vi "samyoung_pm_ZOU.vi"() -> ()   [LabVIEW 2015]
uses:
  <vilib>/DAQmx/read.llb/DAQmx Read.vi
  <vilib>/DAQmx/read.llb/DAQmx Read (Analog DBL 1Chan 1Samp).vi
  <vilib>/DAQmx/create/channels.llb/DAQmx Create Channel (AI-Voltage-Basic).vi
  <vilib>/DAQmx/configure/timing.llb/DAQmx Timing (Sample Clock).vi
  <vilib>/Utility/file.llb/Write To Spreadsheet File (string).vi
  <vilib>/DAQmx/miscellaneous.llb/DAQmx Fill In Error Info.vi
panel:
  in  "Fille Directory":path
  in  "error in":errorcluster
  in  "samples per channel":i32=1000
  in  "rate":dbl=1000.0 format="%0.2f"
  in  "stop":bool
  # "Dust and Gas Sensor Module Output"
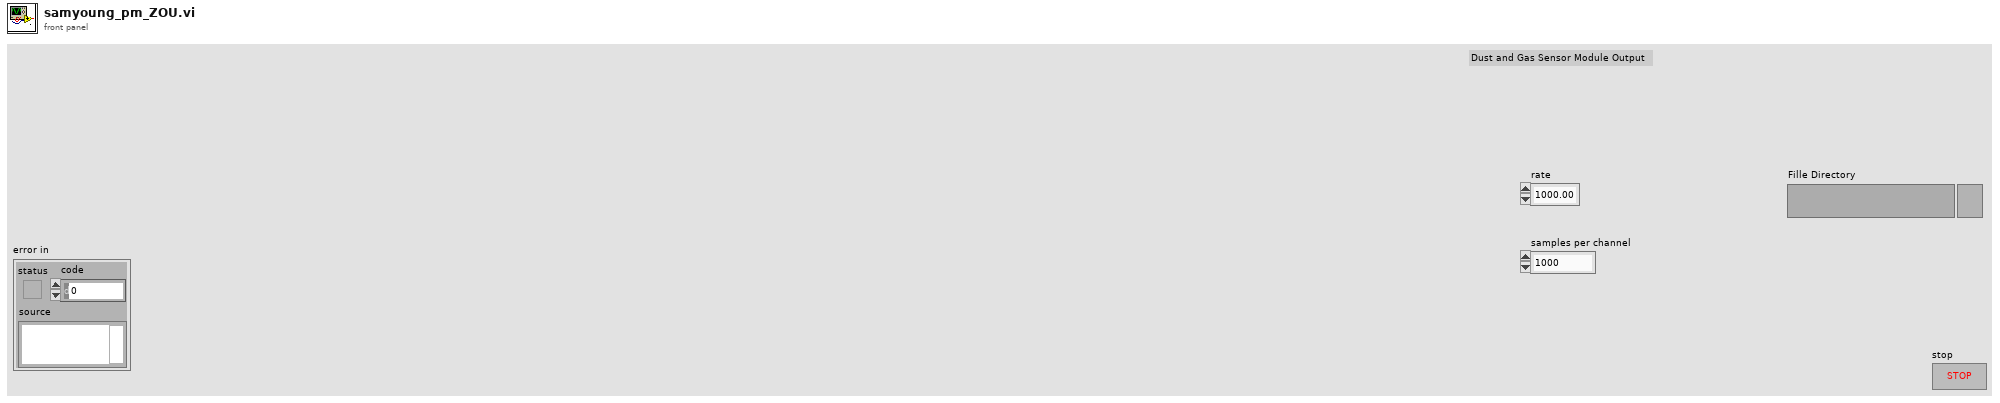
[diagram p1: front panel]
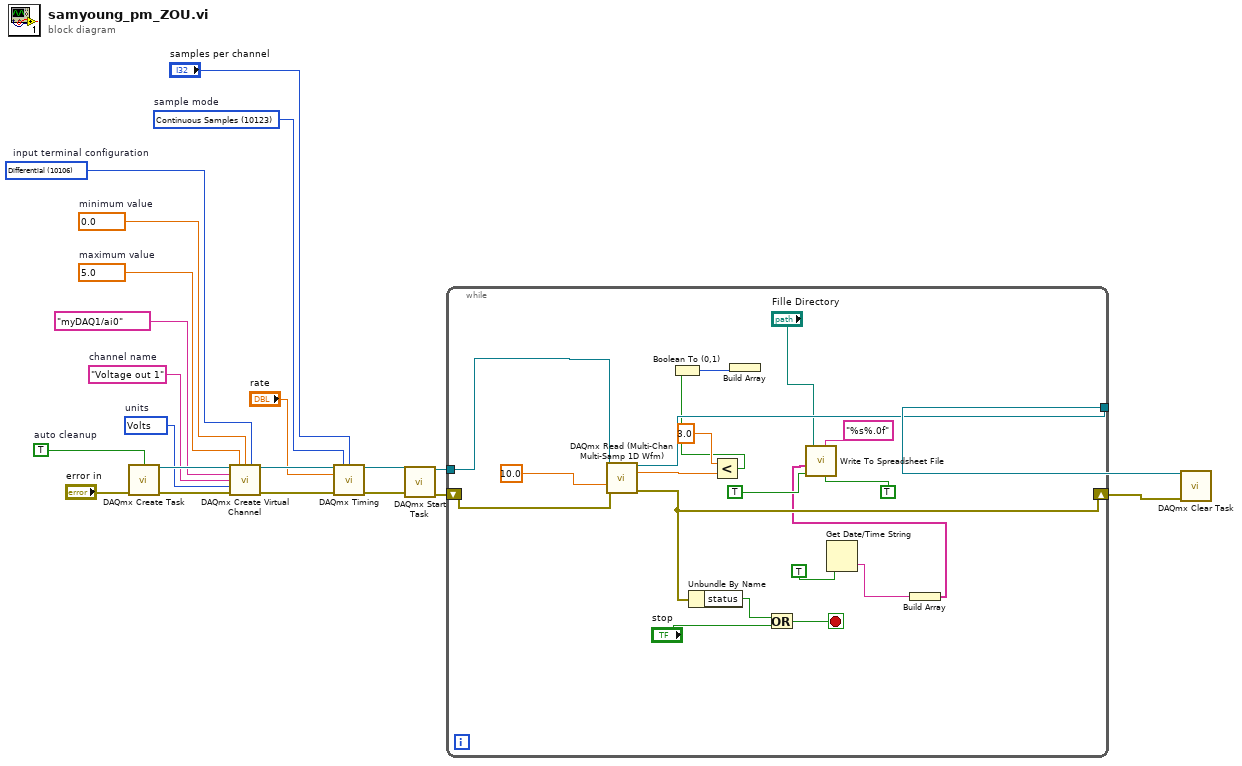
[diagram p0: block diagram]
diagram:
  w6 = 10123 items=["Finite Samples"=10178, "Continuous Samples"=10123, "Hardware Timed Single Point"=12522]  # sample mode
  w8 = 10106 items=["default"=-1, "RSE"=10083, "NRSE"=10078, "Differential"=10106, "Pseudodifferential"=12529]  # input terminal configuration
  w9 = 10348 items=["Volts"=10348, "From Custom Scale"=10065]  # units
  w10 = "Voltage out 1"  # channel name
  w12 = 0.0  # minimum value
  w13 = 5.0  # maximum value
  w15 = TRUE  # auto cleanup
  n1 = call <vilib>:"DAQmx Create Task.vi"("auto cleanup"=w15, "error in"="error in") -> ("task out"=w14:refnum<k21>, "error out"=w16:errorcluster)  [unwired: 12 in]
  n2 = call-poly <vilib>:"DAQmx Create Virtual Channel.vi"("task in"=w14, "maximum value"=w13, "minimum value"=w12, "input terminal configuration"=w8, "physical channels"=tag "myDAQ1/ai0", "name to assign"=w10, "units"=w9, "error in"=w16) -> ("task out"=w7:refnum<k21>, "error out"=w11:errorcluster)  [unwired: 6 in]
  n3 = call-poly <vilib>:"DAQmx Timing.vi"("task/channels in"=w7, "sample mode"=w6, "samples per channel"="samples per channel", "rate"="rate", "error in"=w11) -> ("task out"=w5:refnum<k21>, "error out"=w4:errorcluster)  [unwired: 9 in]
  n4 = call <vilib>:"DAQmx Start Task.vi"("task/channels in"=w5, "error in"=w4) -> ("task out"=w18:refnum<k21>, "error out"=w19:errorcluster)  [unwired: 12 in]
  n5 = while {
    tunnel: w18 -> [w25]
    tunnel: [w39] -> w21
    shift-right: [w37] -> w20
    shift-left: w19 -> [w40]
    stop <- w36 stop-if-true
    n6 = call-poly "DAQmx Read (Multi-Chan Multi-Samp 1D Wfm).vi"("task/channels in"=w25, "timeout"=10.0, "error in"=w40) -> ("task out"=w39:refnum<k21>, "data"=w28:dbl, "error out"=w37:errorcluster)  [unwired: 10 in]
    n7 = Unbundle By Name(w37) -> ("status"=w38:bool)
    n8 = Less?(x=3.0 ("y"), y=w28) -> (x < y?=w27:bool)
    n9 = Boolean To (0,1)(Boolean=w27) -> (0, 1=w30:i16)
    n10 = Build Array(w30) -> ()  [unwired: 1 out]
    n11 = Or(x=w38, y="stop") -> (x .or. y?=w36:bool)
    n12 = Get Date/Time String(want seconds? (F)=TRUE) -> (time string=w23:string)  [unwired: 2 in, 1 out]
    n13 = Build Array(w23) -> (w22:string[])
    n14 = call-poly <vilib>:"Write To Spreadsheet File.vi"("transpose? (no:F)"=TRUE, "format (%s)"="%s%.0f" ("format (%.3f)"), "append to file? (new file:F)"=TRUE, "1D data"=w22, "file path (dialog if empty)"="Fille Directory") -> ()  [unwired: 3 in, 1 out]
  }
  n15 = call <vilib>:"DAQmx Clear Task.vi"("task in"=w21, "error in"=w20) -> ()  [unwired: 13 in, 1 out]
